vi "FTW-CodeGen-GetErrors.vi"(0 "State In":T2 {"Actor Interface"."Bounds"."Left" format="%dpx"; "Actor Interface"."Bounds"."Top" format="%dpx"; "Actor Interface"."Bounds"."Right" format="%dpx"; "Actor Interface"."Bounds"."Bottom" format="%dpx"}, 5 "XRef":refnum<vi>, 7 "Generate Strings?":bool) -> (4 "Errors":T1(array[cluster]), 6 "Errors Present?":bool)   [LabVIEW 2015, in "FTW-Actor-Spawn.xnode"]
uses:
  FTW-Actor-Spawn.xnode
  FTW-CodeGen-State.ctl
panel:
  # "Inputs"
  # "Outputs"
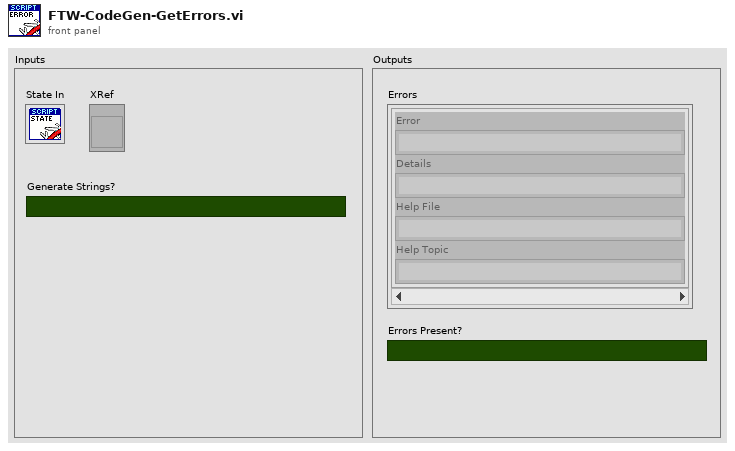
[diagram p1: front panel]
types:
  T1 = cluster{"Error":string, "Details":string, "Help File":string, "Help Topic":string}[]
  T2 = typedef "FTW-Actor-Spawn.xnode/FTW-CodeGen-State.ctl" = cluster{"Path Wired?":bool, "Actor Interface":cluster{"Name":string, "Type":variant, "Bounds":cluster{"Left":i32, "Top":i32, "Right":i32, "Bottom":i32}, "Input":bool, "Recommended":bool, "Required":bool, "Dynamic Dispatch":bool, "On Interface":bool, "\"The\" Config Terminal":bool}[], "Config Terminal Index":i32}
  T3 = cluster{"Error":string, "Details":string, "Help File":string, "Help Topic":string}
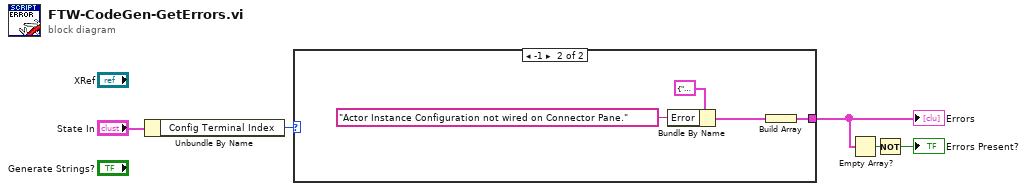
[diagram p0: block diagram]
diagram:
  n1 = Unbundle By Name("State In") -> ("Config Terminal Index"=w4:i32)
  n2 = case shown="-1" w4 {
    tunnel: [_ w7] -> w3
    frame Default {
    }
    frame -1 {
      n3 = Bundle By Name(cluster=T3 {"Error"="", "Details"="", "Help File"="", "Help Topic"=""}, "Error"="Actor Instance Configuration not wired on Connector Pane.") -> (w8:T3)
      n4 = Build Array(w8) -> (w7:T1)
    }
  }
  "Errors" <- w3
  n5 = Empty Array?(array=w3) -> (empty?=w2:bool)
  n6 = Not(x=w2) -> (.not. x?=→"Errors Present?":bool)
